vi "S2C_CMD_ShowMenu.vi"(8 "Error In":errorcluster, 9 "Cell Position":T1, 10 "MenuRef":refnum<k9>, 11 "CtlRef":refnum<vi>) -> (0 "Error Out":errorcluster, 3 "Discard?":bool)   [LabVIEW 2015]
doc: "Loads the popup menu for the selected command input parameter."
uses:
  <vilib>/Utility/miscctls.llb/LVRowAndColumnTypeDef.ctl
  S2C_CMD_Globals.vi
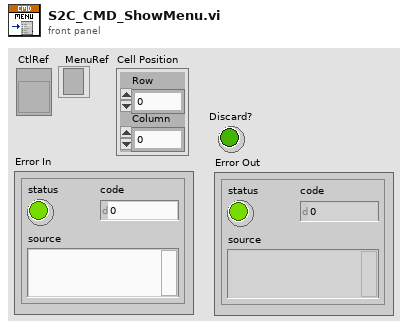
[diagram p1: front panel]
types:
  T1 = typedef "LVRowAndColumnTypeDef.ctl" = cluster{"Row":i32, "Column":i32}
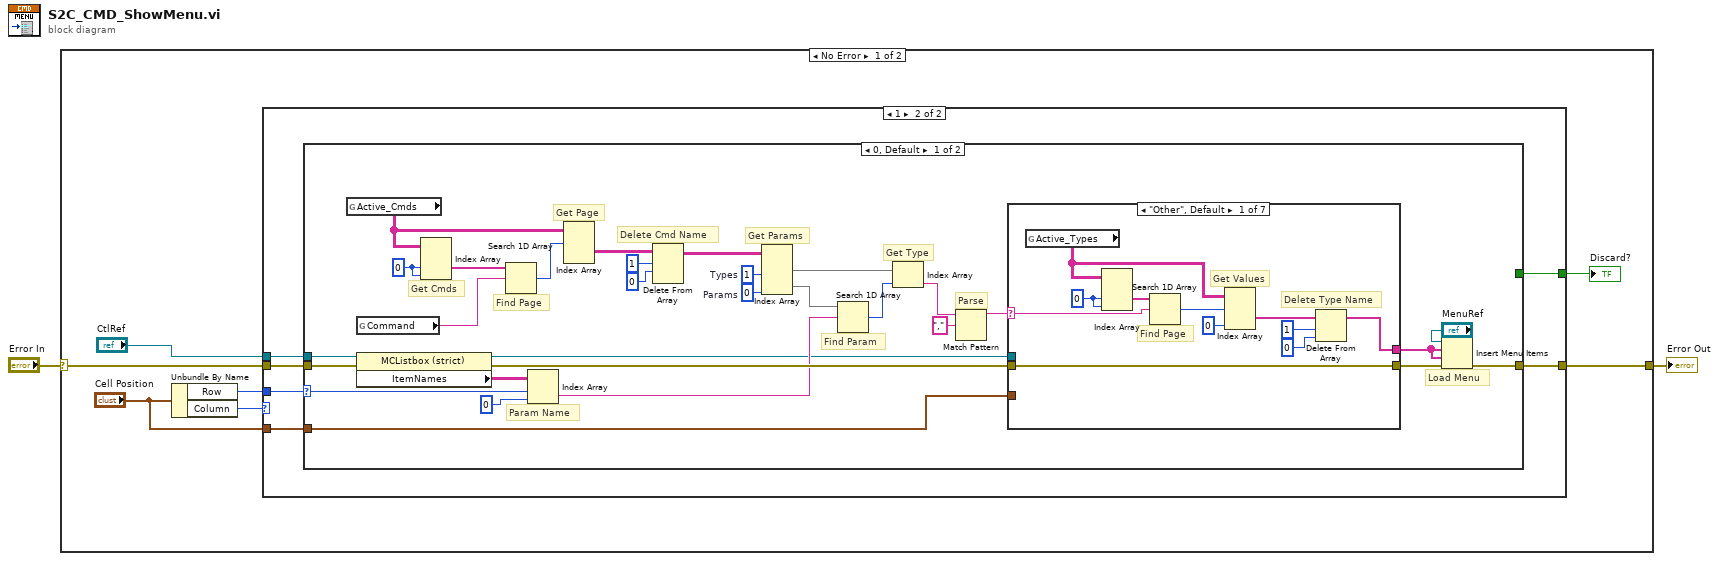
[diagram p0: block diagram]
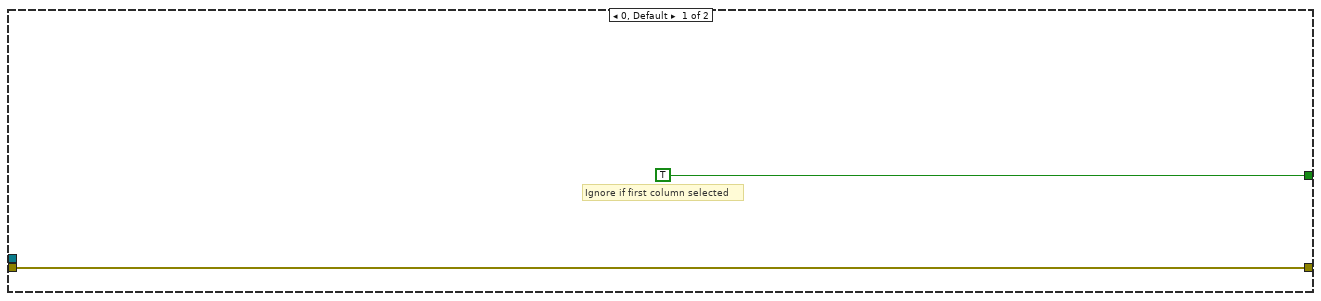
[diagram p2: hidden frame]
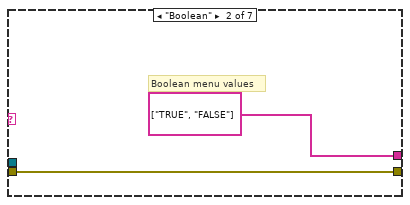
[diagram p3: hidden frame]
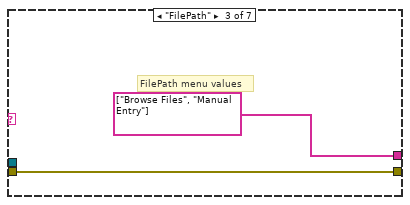
[diagram p4: hidden frame]
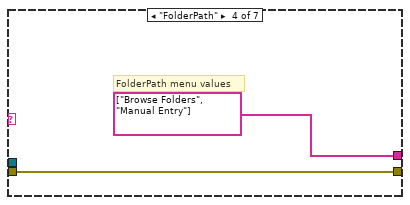
[diagram p5: hidden frame]
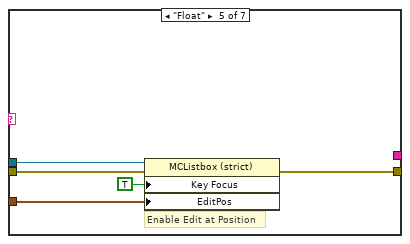
[diagram p6: hidden frame]
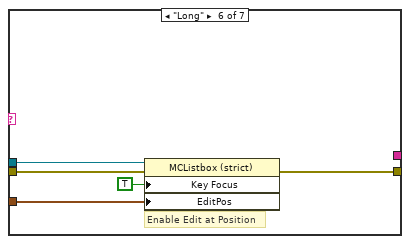
[diagram p7: hidden frame]
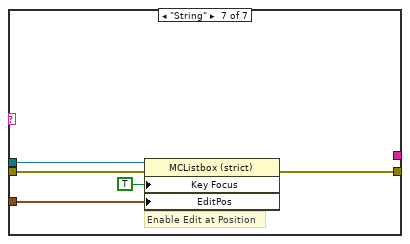
[diagram p8: hidden frame]
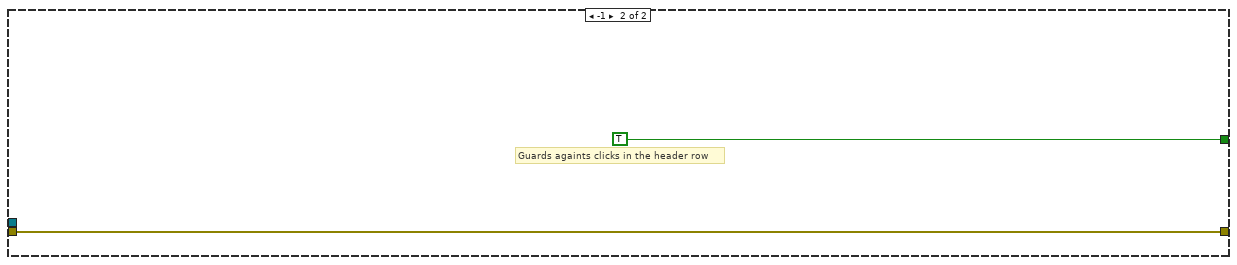
[diagram p9: hidden frame]
diagram:
  n1 = case shown="No Error" "Error In" {
    selector: "Error In" -> [w9 w81]
    tunnel: [w8 w81] -> w1
    frame No Error {
      n2 = Unbundle By Name("Cell Position") -> ("Row"=w7:i32, "Column"=w4:i32)
      n3 = case shown="1" w4 {
        tunnel: w9 -> [w11 w17]
        tunnel: [w11 w16] -> w8
        tunnel: w7 -> [_ w15]
        tunnel: [TRUE w14] -> w6
        tunnel: "Cell Position" -> [_ w13]
        tunnel: "CtlRef" -> [_ w12]
        frame 0, Default {
          # "Ignore if first column selected"
        }
        frame 1 {
          n4 = case shown="0, Default" w15 {
            selector: w15 -> [w41 _]
            tunnel: w17 -> [w43 w80]
            tunnel: [w42 w80] -> w16
            tunnel: [_ TRUE] -> w14
            tunnel: w13 -> [w27 _]
            tunnel: w12 -> [w26 _]
            frame 0, Default {
              w35 = 0  # Params
              w36 = 1  # Types
              w39 = 0 ("disabled index (row)")
              # "Delete Cmd Name"
              # "Parse"
              # "Load Menu"
              # "Get Type"
              # "Find Param"
              # "Get Params"
              # "Get Page"
              # "Find Page"
              # "Get Cmds"
              # "Param Name"
              n5 = global read "S2C_CMD_Globals.vi" "Active_Cmds"() -> (w25:string[][][])
              n6 = global read "S2C_CMD_Globals.vi" "Command"() -> (w38:string)
              n7 = property on="Property Node" class="MCListbox (strict)"(reference=w26, error in=w43) -> (reference out=w28:refnum<vi>, error out=w44:errorcluster, "ItemNames"=w46:string[][])
              n8 = Index Array(array=w25, index (dim 1)=w39, index (dim 2)=w39) -> (element=w40:string[])  [unwired: 1 in]
              n9 = Search 1D Array(1D array=w40, element=w38) -> (index of element=w37:i32)  [unwired: 1 in]
              n10 = Index Array(array=w46, index (row)=w41, index (col)=0 ("disabled index (col)")) -> (element=w31:string)
              n11 = Index Array(array=w25, index (dim 0)=w37) -> (element=w20:string[][])  [unwired: 2 in]
              n12 = Delete From Array(array=w20, length=1, index (row)=0 ("index")) -> (array with subset deleted=w18:string[][])  [unwired: 1 in, 1 out]
              n13 = Index Array(array=w18, index (col) #1=w36, index (col) #2=w35) -> (element #1=w33:string[], element #2=w34:string[])  [unwired: 2 in]
              n14 = Search 1D Array(1D array=w34, element=w31) -> (index of element=w32:i32)  [unwired: 1 in]
              n15 = Index Array(array=w33, index=w32) -> (element=w24:string)
              n16 = Match Pattern(string=w24, regular expression=",") -> (before substring=w22:string)  [unwired: 1 in, 3 out]
              n17 = case shown="\"Other\", Default" w22 {
                selector: w22 -> [w50 _ _ _ _ _ _]
                tunnel: w44 -> [w49 w59 w61 w63 w67 w72 w77]
                tunnel: [w49 w59 w61 w63 w66 w71 w76] -> w42
                tunnel: [w48 string[] ["TRUE", "FALSE"] string[] ["Browse Files", "Manual Entry"] string[] ["Browse Folders", "Manual Entry"] _ _ _] -> w29
                tunnel: w28 -> [_ _ _ _ w65 w70 w75]
                tunnel: w27 -> [_ _ _ _ w64 w69 w74]
                frame "Other", Default {
                  w57 = 0 ("disabled index (row)")
                  # "Delete Type Name"
                  # "Get Values"
                  # "Find Page"
                  n18 = global read "S2C_CMD_Globals.vi" "Active_Types"() -> (w47:string[][][])
                  n19 = Index Array(array=w47, index (dim 1)=w57, index (dim 2)=w57) -> (element=w56:string[])  [unwired: 1 in]
                  n20 = Search 1D Array(1D array=w56, element=w50) -> (index of element=w55:i32)  [unwired: 1 in]
                  n21 = Index Array(array=w47, index (dim 0)=w55, index (dim 2)=0 ("disabled index (col)")) -> (element=w53:string[])  [unwired: 1 in]
                  n22 = Delete From Array(array=w53, length=1, index=0) -> (array with subset deleted=w48:string[])  [unwired: 1 out]
                }
                frame "Boolean" {
                  # "Boolean menu values"
                }
                frame "FilePath" {
                  # "FilePath menu values"
                }
                frame "FolderPath" {
                  # "FolderPath menu values"
                }
                frame "Float" {
                  # "Enable Edit at Position"
                  n23 = property on="Property Node" class="MCListbox (strict)"(reference=w65, error in=w67, "Key Focus"=TRUE, "EditPos"=w64) -> (error out=w66:errorcluster)  [unwired: 1 out]
                }
                frame "Long" {
                  # "Enable Edit at Position"
                  n24 = property on="Property Node" class="MCListbox (strict)"(reference=w70, error in=w72, "Key Focus"=TRUE, "EditPos"=w69) -> (error out=w71:errorcluster)  [unwired: 1 out]
                }
                frame "String" {
                  # "Enable Edit at Position"
                  n25 = property on="Property Node" class="MCListbox (strict)"(reference=w75, error in=w77, "Key Focus"=TRUE, "EditPos"=w74) -> (error out=w76:errorcluster)  [unwired: 1 out]
                }
              }
              n26 = Insert Menu Items(7:w29, 8:w29, 9:"MenuRef") -> ()  [unwired: 3 in, 3 out]
            }
            frame -1 {
              # "Guards againts clicks in the header row"
            }
          }
        }
      }
      "Discard?" <- w6
    }
    frame Error {
    }
  }
  "Error Out" <- w1
